vi "Force reset.vi"(7 "Timeout (100 ms)":i32=100, 8 "Error In":errorcluster, 10 "Reset Target":u8[](array[numeric]), 11 "LINX Device Config":T1) -> (0 "Error Out":errorcluster, 3 "Dup LINX Device Config":T1)   [LabVIEW 2019, in "LINXx.lvlib"]
doc: "Resets board or one of its communication links."
uses:
  LINXx.lvlib
  <vilib>/MakerHub/LINX/Private/Device/Type Defs/LINX Device Config.ctl
  <vilib>/MakerHub/LINX/Private/Type Defs/Interface.ctl
  <vilib>/MakerHub/LINX/Private/Device/Type Defs/TCP Config.ctl
  <vilib>/MakerHub/LINX/Private/Device/Type Defs/Channels.ctl
  <vilib>/MakerHub/LINX/Private/Type Defs/Error Type.ctl
  <vilib>/MakerHub/LINX/Private/Device/Device.lvlib
  <vilib>/MakerHub/LINX/LMH-LINX.lvlib
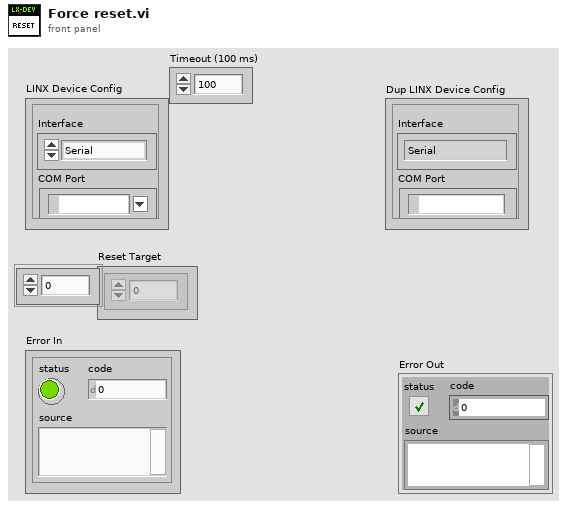
[diagram p1: front panel]
types:
  T1 = typedef "LMH-LINX.lvlib/Device.lvlib/LINX Device Config.ctl" = cluster{"Interface":T2, "COM Port":refnum<visa-resource-name>, "TCP Configuration":T3, "Device Family":u8, "Device ID":u8, "Device Name":string, "TCP Ref":refnum<k5>, "Channels":T4}
  T2 = typedef "LMH-LINX.lvlib/Interface.ctl" = enum16{"Serial", "TCP"}
  T3 = typedef "LMH-LINX.lvlib/Device.lvlib/TCP Config.ctl" = cluster{"IP Address":string, "Port":u16}
  T4 = typedef "LMH-LINX.lvlib/Channels.ctl" = cluster{"DI":u8[], "DO":u8[], "AI":u8[], "AO":u8[], "PWM":u8[], "QE":u8[], "UART":u8[], "I2C 2":u8[], "SPI":u8[], "CAN":u8[], "Servo":u8[], "AI Ref (V)":dbl, "AI Resolution (Bits)":u8, "AO Ref (V)":dbl, "AO Resolution (Bits)":u8}
  T5 = typedef "LMH-LINX.lvlib/Error Type.ctl" = enum16{"Unknown", "Timeout", "Corrupt Return Packet", "Unable To Connect", "Command Not Supported", "Channel DNE", "Invalid COM Config", "Firmware Version Mismatch", "myRIO Support", "CMD Specific Error", "Local IO Not Supported"}
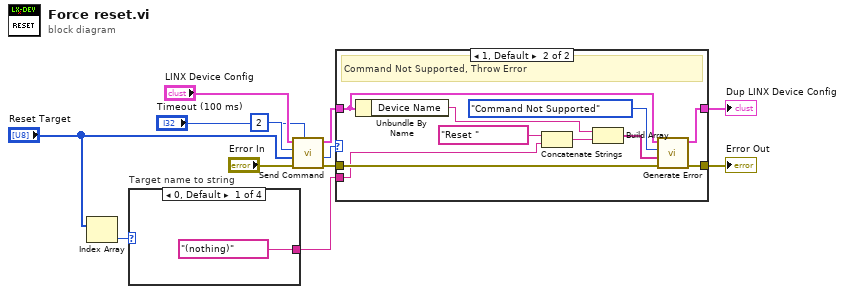
[diagram p0: block diagram]
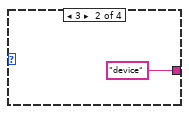
[diagram p2: hidden frame]
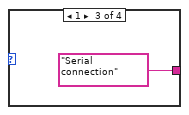
[diagram p3: hidden frame]
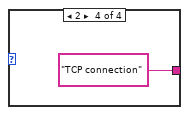
[diagram p4: hidden frame]
diagram:
  n1 = Index Array(array="Reset Target") -> (element=w3:u8)  [unwired: 1 in]
  n2 = case "Target name to string" shown="0, Default" w3 {
    tunnel: ["(nothing)" "device" "Serial connection" "TCP connection"] -> w2
    frame 0, Default {
    }
    frame 3 {
    }
    frame 1 {
    }
    frame 2 {
    }
  }
  n3 = call <vilib>:"Send Command.vi"("Timeout (100 ms)"="Timeout (100 ms)", "Error In"="Error In", "ARGS"="Reset Target", "CMD"=u16 2, "LINX Device Config"="LINX Device Config") -> ("Error Out"=w8:errorcluster, "Status"=w11:u8, "LINX Device Config"=w7:T1)  [unwired: 3 in, 1 out]
  n4 = case shown="1, Default" w11 {
    tunnel: w8 -> [w17 w25]
    tunnel: w7 -> [w18 w21]
    tunnel: [w18 w23] -> w5
    tunnel: [w17 w22] -> w6
    tunnel: w2 -> [_ w19]
    frame 0 {
      # "ok"
    }
    frame 1, Default {
      # "Command Not Supported, Throw Error"
      n5 = Unbundle By Name(w21) -> ("Device Name"=w27:string)
      n6 = Concatenate Strings("Reset ", w19) -> (w20:string)
      n7 = Build Array(w27, w20) -> (w28:string[])
      n8 = call <vilib>:"Generate Error.vi"("Error In"=w25, "Arguments"=w28, "Error Type"=Error_Type."Command Not Supported", "LINX Device Config"=w21) -> ("Error Out"=w22:errorcluster, "Dup LINX Device Config"=w23:T1)  [unwired: 6 in]
    }
  }
  "Error Out" <- w6
  "Dup LINX Device Config" <- w5
